vi "Emballage_BDD_chargement_IDArticle_GPAO.vi"(2 "Refnum Ch":refnum<vi>, 5 "entrée d'erreur (pas d'erreur)":errorcluster, 8 "progress":refnum<vi>) -> (16 "Tableau en sortie":string[][](array[string]), 19 "sortie d'erreur":errorcluster)   [LabVIEW 2020]
uses:
  Modules/FS/60_FS_Controles/60_FS_SetGet.ctl
panel:
  out "Suffixe":string
  out "Longeur_No_Serie":string
  out "code_barre_fixe_fin":string
  out "date":string
  out "Famille":string
  out "ID":string
  out "tableau ajouté":string[](array[string])
  out "INDICE_REV":string
  out "id_article":string
  out "clc_designation":string
  out "suffixe":string
  out "codification":string
  out "Indice":string
  out "Code_Barre_Fixe":string
  out "Nb_valve_par_carton":string
  out "melange_des_lots_possible":string
  out "affiche_code_barre_client":string
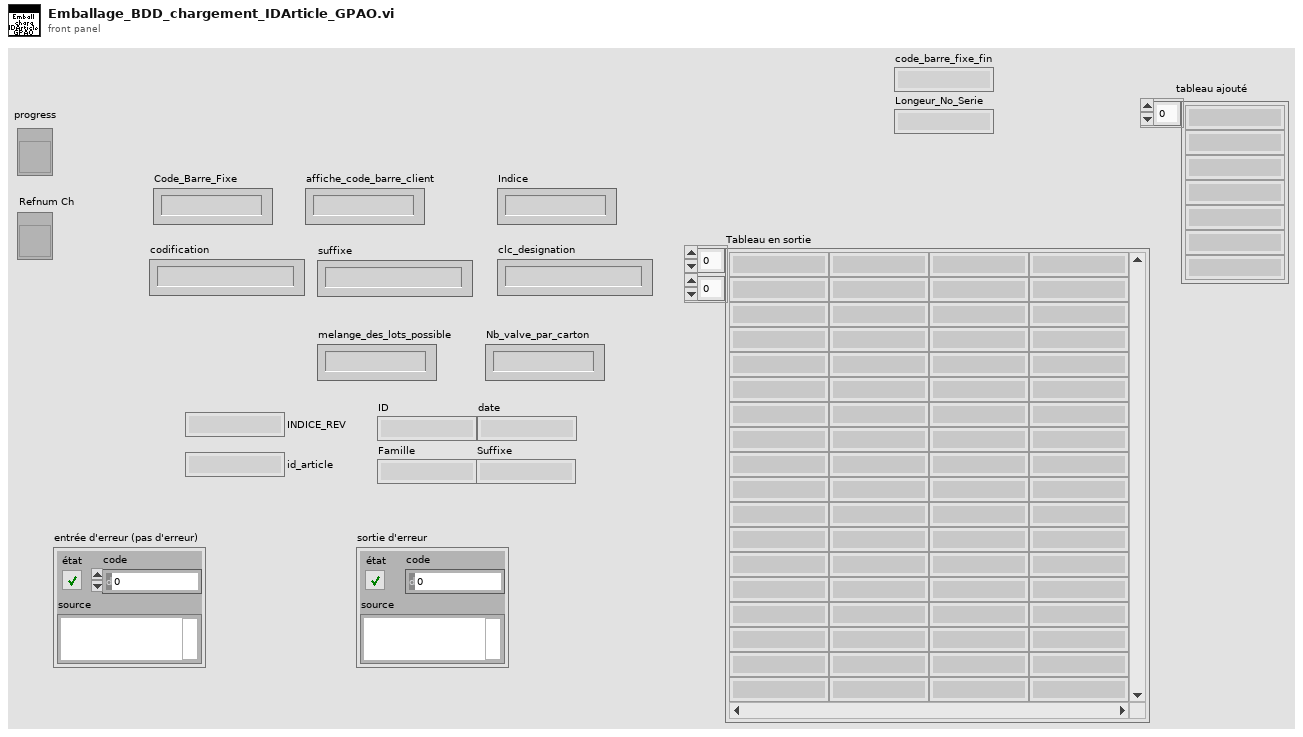
[diagram p1: front panel]
types:
  T1 = typedef "60_FS_SetGet.ctl" = enum16{"set", "get"}
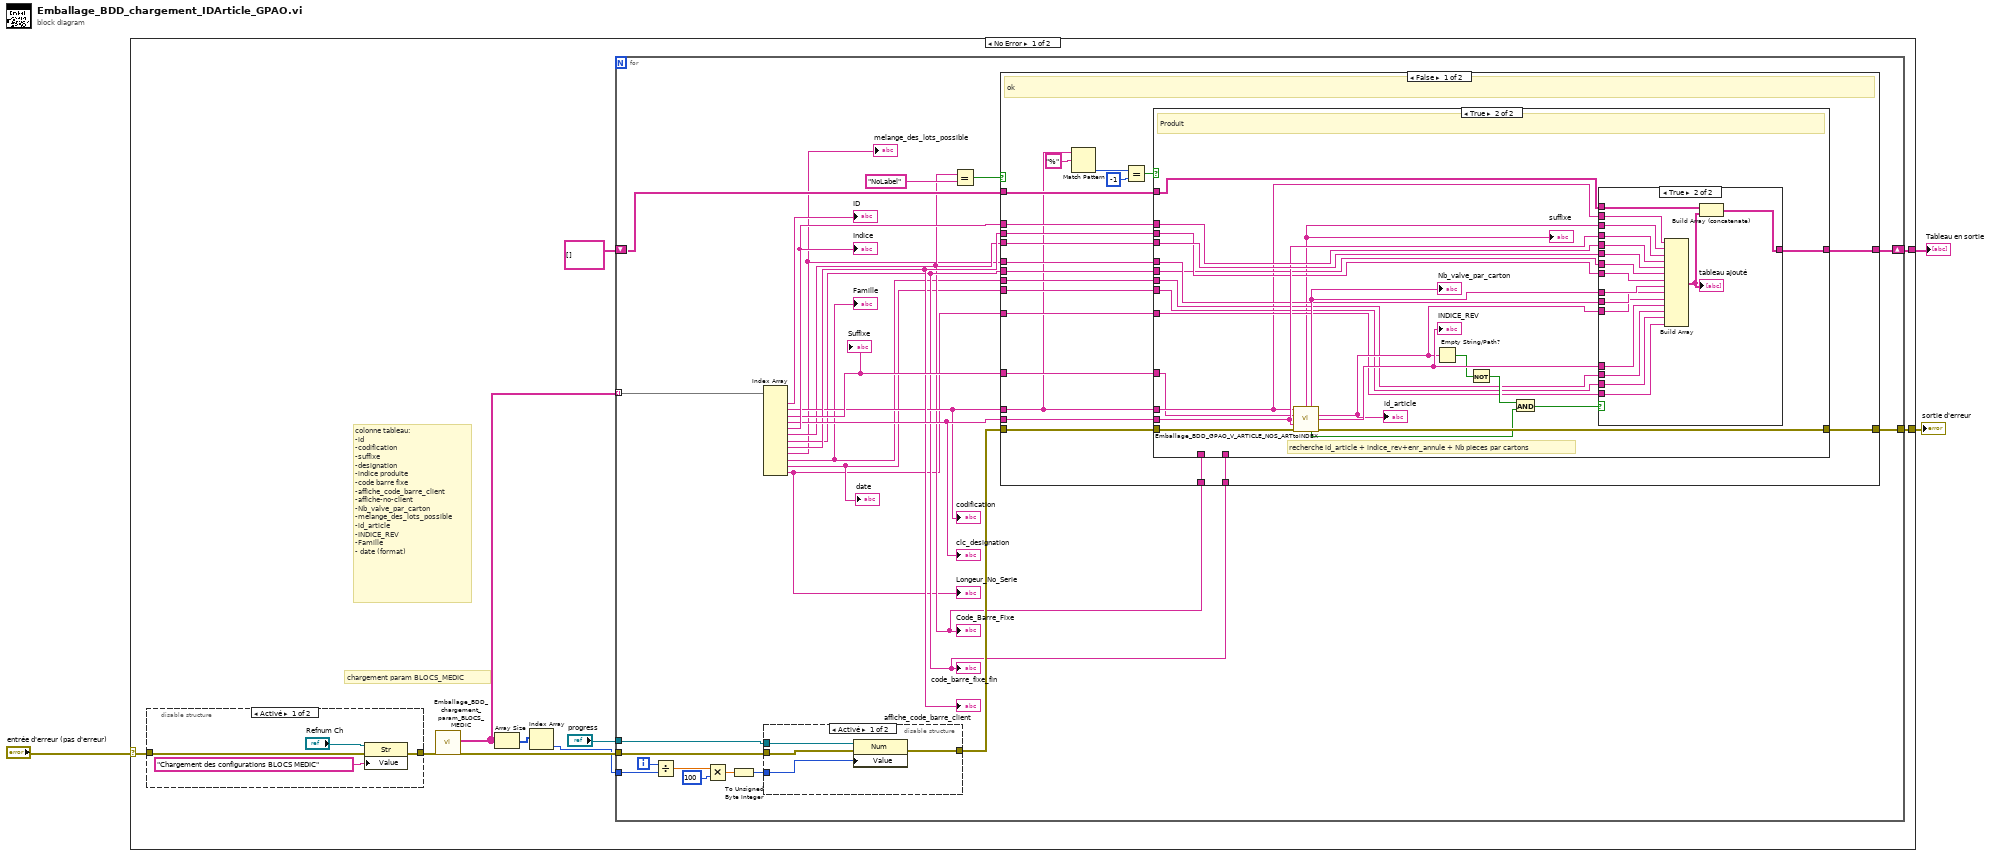
[diagram p0: block diagram]
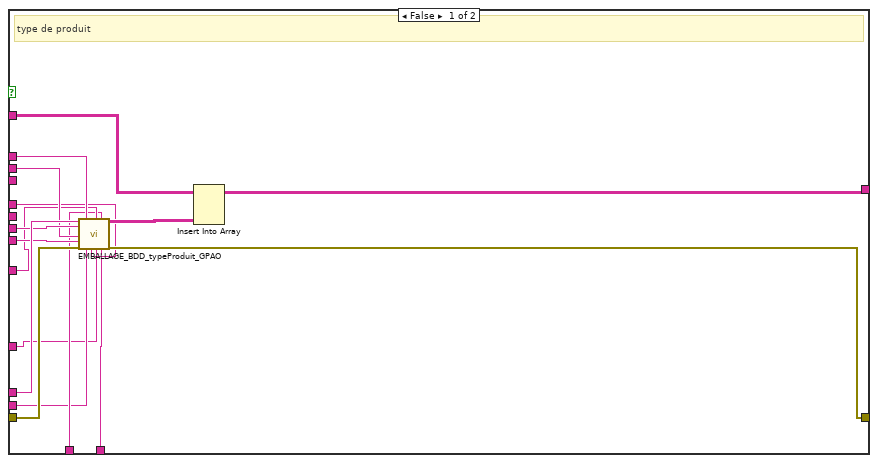
[diagram p3: hidden frame]
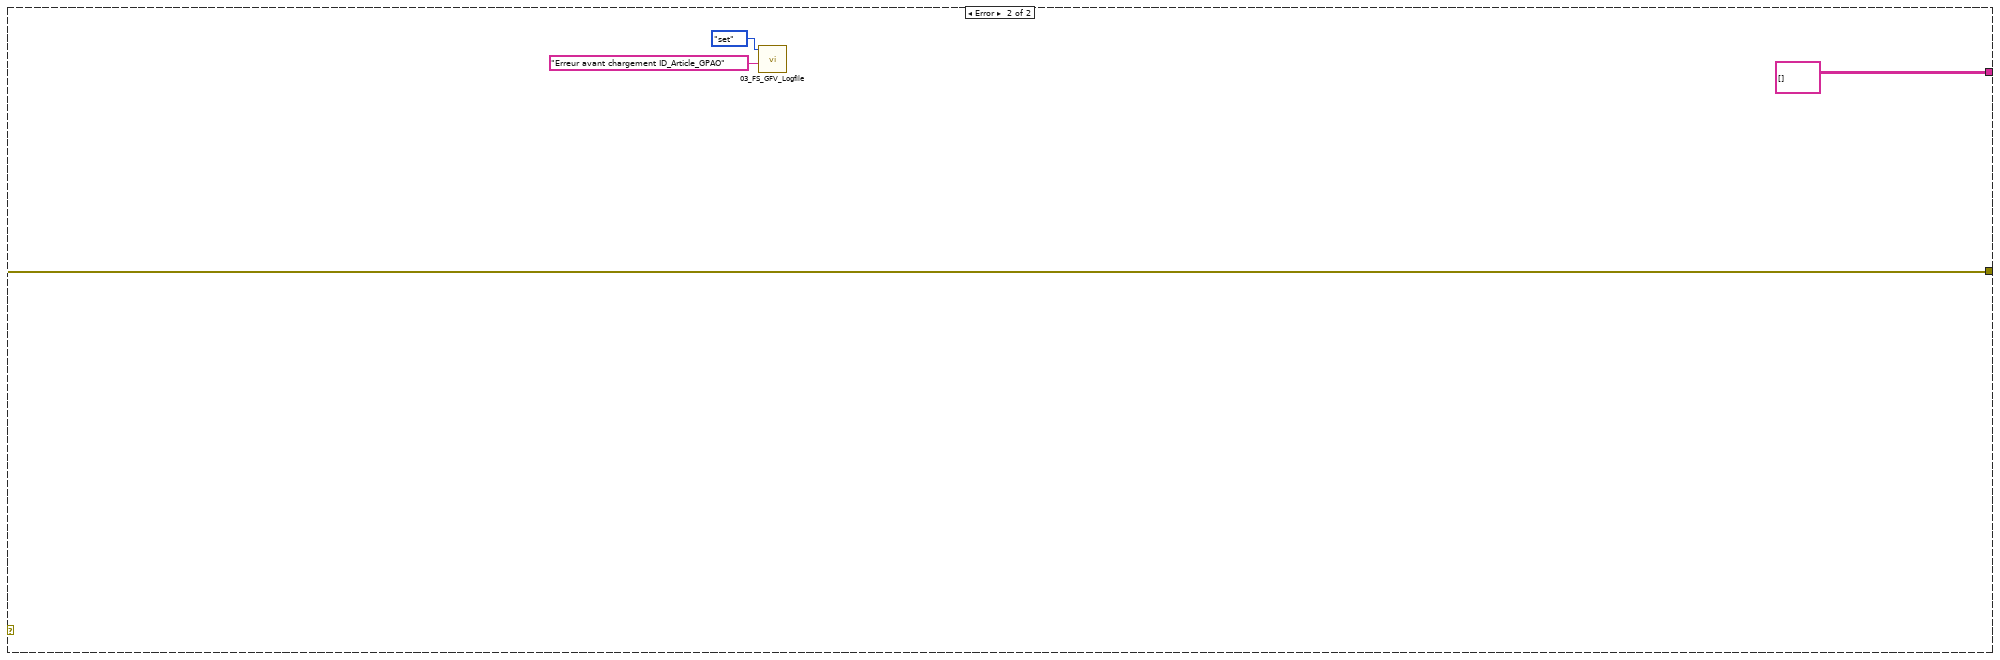
[diagram p7: hidden frame]
diagram:
  n1 = case shown="No Error" "entrée d'erreur (pas d'erreur)" {
    selector: "entrée d'erreur (pas d'erreur)" -> [w10 w134]
    tunnel: [w13 string[][] [] ("Tableau en entrée")] -> w3
    tunnel: [w11 w134] -> w1
    frame No Error {
      # "colonne tableau:\n-id\n-codification\n-suffixe\n-designation\n-indice produite\n-code barre fixe\n-affiche_code_barre_client\n-affiche-no-client\n-Nb_valve_par_carton\n-melange_des_lots_possible\n-id_article\n-INDICE_REV\n-Famille\n- date (format)"
      # "chargement param BLOCS_MEDIC"
      n2 = disable-structure shown="Activé" {
        disable-tunnel: w10 -> [w15 w18]
        disable-tunnel: [w14 w18] -> w8
        frame Enabled {
          n3 = property class="Str"(reference="Refnum Ch", error in=w15, "Value"="Chargement des configurations BLOCS MEDIC" ("Valeur")) -> (error out=w14:errorcluster)  [unwired: 1 out]
        }
        frame Disabled {
        }
      }
      n4 = call "Emballage_BDD_chargement_param_BLOCS_MEDIC.vi"("Error in"=w8) -> ("Error out"=w7:errorcluster, "Result Set"=w6:string[][])  [unwired: 8 in, 1 out]
      n5 = Array Size(array=w6) -> (size(s)=w5:i32[])
      n6 = Index Array(array=w5) -> (element=w4:i32)  [unwired: 1 in]
      n7 = for {
        tunnel: w6 -> [w33] mode=indexing
        tunnel: w7 -> [w36]
        tunnel: w4 -> [w41]
        shift-right: [w39] -> w13
        shift-left: string[][] [] ("Tableau en entrée") -> [w40]
        tunnel: [w37] -> w11
        tunnel: "progress" -> [w35]
        i -> [w42]
        n8 = Divide(x=w42, y=w41) -> (x/y=w43:dbl)
        n9 = Multiply(x=w43, y=u8 100) -> (x*y=w45:dbl)
        n10 = To Unsigned Byte Integer(number=w45) -> (unsigned 8bit integer=w38:u8)
        n11 = Index Array(array=w33) -> (element #1=→"ID":string, element #2=w27:string, element #3=w29:string, element #4=w30:string, element #5=w31:string, element #6=w23:string, element #7=w24:string, element #8=w28:string, element #9=w22:string, element #10=w21:string, element #11=w20:string, element #12=w19:string)  [unwired: 12 in]
        "affiche_code_barre_client" <- w28
        "melange_des_lots_possible" <- w22
        "Code_Barre_Fixe" <- w23
        "Indice" <- w31
        "codification" <- w27
        "clc_designation" <- w30
        "Famille" <- w21
        "code_barre_fixe_fin" <- w24
        "date" <- w20
        "Longeur_No_Serie" <- w19
        "Suffixe" <- w29
        n12 = disable-structure shown="Activé" {
          disable-tunnel: w38 -> [w129 _]
          disable-tunnel: w36 -> [w128 w130]
          disable-tunnel: w35 -> [w127 _]
          disable-tunnel: [w126 w130] -> w34
          frame Enabled {
            n13 = property class="Num"(reference=w127, error in=w128, "Value"=w129) -> (error out=w126:errorcluster)  [unwired: 1 out]
          }
          frame Disabled {
          }
        }
        n14 = Equal?(x=w23, y="NoLabel") -> (x = y?=w26:bool)
        n15 = case shown="False" w26 {
          tunnel: w40 -> [w66 w125]
          tunnel: [w65 w125] -> w39
          tunnel: [w64 w124] -> w37
          tunnel: w34 -> [w63 w124]
          tunnel: w31 -> [w62 _]
          tunnel: w23 -> [w61 _]
          tunnel: w30 -> [w60 _]
          tunnel: w29 -> [w59 _]
          tunnel: w20 -> [w58 _]
          tunnel: w21 -> [w57 _]
          tunnel: w22 -> [w56 _]
          tunnel: w28 -> [w55 _]
          tunnel: w24 -> [w54 _]
          tunnel: w19 -> [w53 _]
          tunnel: w27 -> [w48 _]
          tunnel: w24 -> [w47 _]
          tunnel: w23 -> [w46 _]
          frame False {
            # "ok"
            n16 = Match Pattern(string=w48, regular expression="%" ("expression régulière")) -> (offset past match=w52:i32)  [unwired: 1 in, 3 out]
            n17 = Equal?(x=w52, y=-1) -> (x = y?=w49:bool)
            n18 = case shown="True" w49 {
              tunnel: w66 -> [w78 w104]
              tunnel: [w77 w103] -> w65
              tunnel: [w81 w102] -> w64
              tunnel: w63 -> [w82 w95]
              tunnel: w62 -> [w73 w94]
              tunnel: w61 -> [_ w93]
              tunnel: w60 -> [w68 w92]
              tunnel: w59 -> [w67 w84]
              tunnel: w58 -> [w75 w91]
              tunnel: w57 -> [w79 w90]
              tunnel: w56 -> [w71 w89]
              tunnel: w55 -> [w74 w88]
              tunnel: w54 -> [_ w87]
              tunnel: w53 -> [w72 w86]
              tunnel: w48 -> [w80 w85]
              tunnel: w47 -> [w70 _]
              tunnel: w46 -> [w69 _]
              frame False {
                # "type de produit"
                n19 = call "EMBALLAGE_BDD_typeProduit_GPAO.vi"("NOS_ARTICLE(%)"=w80, "Famille"=w79, "affiche code barre client"=w74, "date"=w75, "error in (no error)"=w82, "indice_produit"=w73, "clc_designation"=w68, "Mélange_lots_possible"=w71, "longeur_No_série"=w72, "SUFFIXE"=w67, "Code_barre_fixe"=w69, "Code_barre_fixe_fin"=w70) -> ("Tableau"=w76:string[][], "error out"=w81:errorcluster)  [unwired: 6 in]
                n20 = Insert Into Array(array=w78, new element=w76) -> (w77:string[][])  [unwired: 2 in]
              }
              frame True {
                # "recherche id_article + indice_rev+enr_annule + Nb pieces par cartons"
                # "Produit"
                n21 = call "Emballage_BDD_GPAO_V_ARTICLE_NOS_ARTtoINDEX.vi"("codification"=w85, "suffixe"=w84, "clc_designation"=w92, "error in (no error)"=w95) -> ("SUFFIXE"=w83:string, "NB_PIECE_EMB"=w100:string, "id_article"=w98:string, "INDICE_REV"=w105:string, "pce_non_annule"=w101:bool, "error out"=w102:errorcluster)  [unwired: 4 in, 2 out]
                "Nb_valve_par_carton" <- w100
                "suffixe" <- w83
                "id_article" <- w98
                "INDICE_REV" <- w105
                n22 = Empty String/Path?(string/path=w98) -> (empty?=w97:bool)
                n23 = Not(x=w97) -> (.not. x?=w96:bool)
                n24 = And(x=w96, y=w101) -> (x .and. y?=w99:bool)
                n25 = case shown="True" w99 {
                  tunnel: w85 -> [_ w123]
                  tunnel: w83 -> [_ w122]
                  tunnel: w92 -> [_ w121]
                  tunnel: w94 -> [_ w120]
                  tunnel: w93 -> [_ w119]
                  tunnel: w88 -> [_ w118]
                  tunnel: w100 -> [_ w117]
                  tunnel: w89 -> [_ w116]
                  tunnel: w98 -> [_ w115]
                  tunnel: w105 -> [_ w114]
                  tunnel: w104 -> [w106 w113]
                  tunnel: [w106 w112] -> w103
                  tunnel: w90 -> [_ w110]
                  tunnel: w91 -> [_ w109]
                  tunnel: w87 -> [_ w108]
                  tunnel: w86 -> [_ w107]
                  frame False {
                    # "enregistrement annulé\npas afficher"
                  }
                  frame True {
                    n26 = Build Array(w123, w122, w121, w120, w119, w108, w118, w117, w116, w115, w114, w110, w109, w107) -> (w111:string[])
                    "tableau ajouté" <- w111
                    n27 = Build Array (concatenate)(w113, w111) -> (w112:string[][])
                  }
                }
              }
            }
          }
          frame True {
            # "rien faire"
            # "Produit sans étiquette"
          }
        }
      }
    }
    frame Error {
      n28 = call "03_FS_GFV_Logfile.vi"("Chaîne"="Erreur avant chargement ID_Article_GPAO", "States"=60_FS_SetGet."set") -> ()  [unwired: 8 in, 2 out]
    }
  }
  "Tableau en sortie" <- w3
  "sortie d'erreur" <- w1
